vi "Set Destination.vi"(8 "error in (no error)":errorcluster, 9 "Destination label":string, 10 "ProjectItem Refnum":refnum<vi>, 11 "Build in":refnum<class "NI_AB_API_Build.lvclass">) -> (0 "error out":errorcluster, 3 "Build out":refnum<class "NI_AB_API_Build.lvclass">)   [LabVIEW 2020, in "NI_AB_API_Build.lvclass"]
uses:
  <vilib>/AppBuilder/AB_API/Build/NI_AB_API_Build.lvclass
  <vilib>/AppBuilder/AB_API/Build/NI_AB_API_Build.lvclass/NI_AB_API_Build.ctl
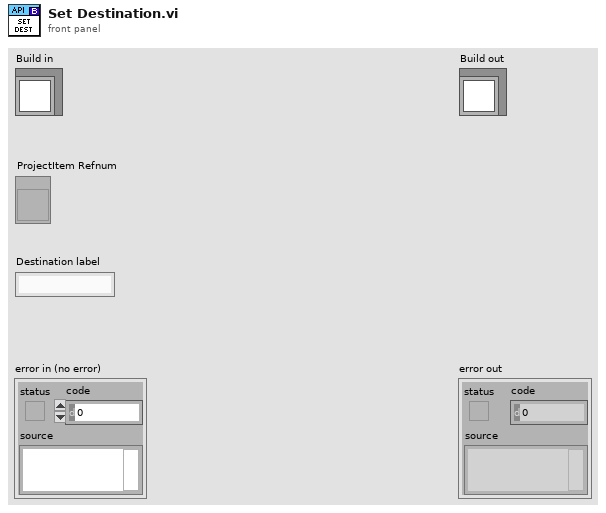
[diagram p1: front panel]
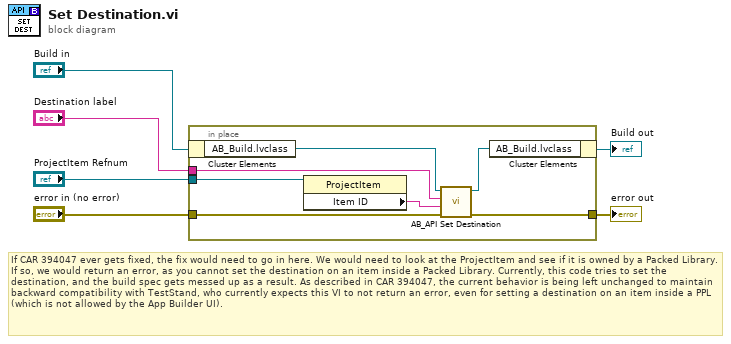
[diagram p0: block diagram]
diagram:
  # "If CAR 394047 ever gets fixed, the fix would need to go in here. We would need to look at the ProjectItem and see if it is owned by a Packed Library. If so, we would return an error, as you cannot set the destination on an item inside a Packed Library. Currently, this code tries to set the destination, and the build spec gets messed up as a result. As described in CAR 394047, the current behavior is being left unchanged to maintain backward compatibility with TestStand, who currently expects this VI to not return an error, even for setting a destination on an item inside a PPL (which is not allowed by the App Builder UI)."
  n1 = in-place {
    in-place-border: "ProjectItem Refnum" -> [w13]
    in-place-border: "Destination label" -> [w12]
    in-place-border: "error in (no error)" -> [w11]
    in-place-border: [w10] -> w5
    n2 = in-place-cluster #1("Build in") -> ("AB_Build.lvclass"=w8:refnum<class "AB_Build.lvclass">)
    n3 = property class="ProjectItem"(reference=w13) -> ("Item ID"=w9:string)  [unwired: 1 in, 2 out]
    n4 = call <vilib>:"AB_API Set Destination.vi"("error in (no error)"=w11, "source item ID"=w9, "Destination label"=w12, "Build in"=w8) -> ("error out"=w10:errorcluster, "Build out"=w7:refnum<class "AB_Build.lvclass">)  [unwired: 6 out]
    n5 = in-place-cluster #1("AB_Build.lvclass"=w7) -> (→"Build out":refnum<class "NI_AB_API_Build.lvclass">)
  }
  "error out" <- w5
